vi "配置变量_temp_赋值.vi"(8 "error in (no error)":errorcluster caption="错误输入（无错误）") -> (0 "error out":errorcluster caption="错误输出")   [LabVIEW 2014]
doc: "该模板用于创建子VI。"
uses:
  glb/glb_data.vi
  R/manifest.vi
  glb/glb_static.vi
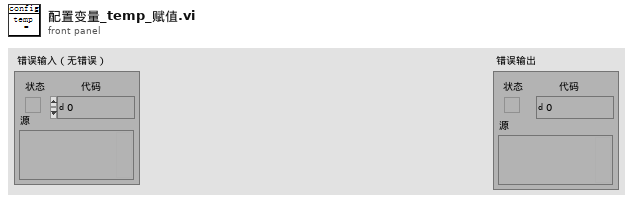
[diagram p1: front panel]
types:
  T1 = cluster{"控制型号":string, "插槽数目":u32, "板卡信息":cluster{"板卡类型":string, "信号类型":string, "上限":string, "下限":string, "单位":string, "通道数":u32, "最大采样率":u32, "设置采样率":u32, "附加条件":string[], "板卡型号":string}[]}
  T2 = cluster{"侧边栏数据":cluster{"来源":string, "名称":string}[], "界面刷间隔率":dbl}
  T3 = cluster{"名称":string, "简称":string, "单位":string, "附加":string[], "类型":enum16{"测试模块", "FPGA", "cRIO", "其他设备", "总体展示"}}[]
  T4 = cluster{"应用状态":bool, "vi名称":string, "刷新间隔":u32, "显示数据精度":u32, "储存数据精度":u32}[]
  T5 = cluster{"应用1":string[], "应用2":string[], "应用3":string[], "应用4":string[], "应用5":string[], "应用6":string[], "应用7":string[], "应用8":string[], "分母":cluster{"来源":string, "名称":string}, "加":cluster{"来源":string, "名称":string}[], "减":cluster{"来源":string, "名称":string}[]}
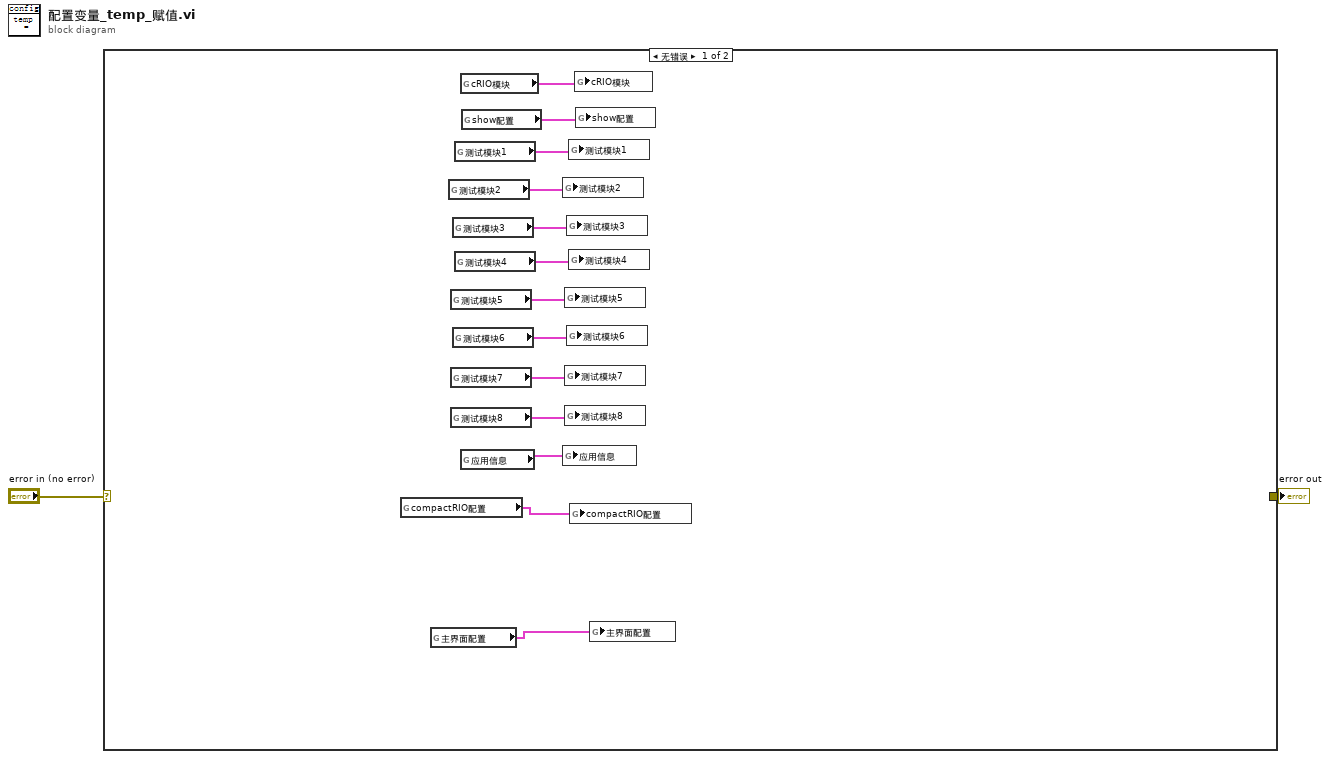
[diagram p0: block diagram]
diagram:
  n1 = case shown="无错误" "error in (no error)" {
    selector: "error in (no error)" -> [_ w16]
    tunnel: [_ w16] -> w1
    frame No Error {
      n2 = global read "glb_static.vi" "compactRIO配置"() -> (w4:T1)
      n3 = global read "glb_static.vi" "主界面配置"() -> (w3:T2)
      n4 = global read "glb_data.vi" "测试模块2"() -> (w8:T3)
      n5 = global read "glb_data.vi" "测试模块5"() -> (w11:T3)
      n6 = global read "glb_data.vi" "测试模块7"() -> (w13:T3)
      n7 = global read "glb_data.vi" "测试模块8"() -> (w14:T3)
      n8 = global read "glb_data.vi" "测试模块3"() -> (w9:T3)
      n9 = global read "glb_data.vi" "测试模块6"() -> (w12:T3)
      n10 = global read "glb_data.vi" "测试模块1"() -> (w7:T3)
      n11 = global read "glb_data.vi" "测试模块4"() -> (w10:T3)
      n12 = global read "glb_data.vi" "cRIO模块"() -> (w5:T3)
      n13 = global read "manifest.vi" "应用信息"() -> (w15:T4)
      n14 = global read "glb_data.vi" "show配置"() -> (w6:T5)
      n15 = global write "配置变量_temp.vi" "测试模块2"(w8) -> ()
      n16 = global write "配置变量_temp.vi" "应用信息"(w15) -> ()
      n17 = global write "配置变量_temp.vi" "测试模块5"(w11) -> ()
      n18 = global write "配置变量_temp.vi" "测试模块7"(w13) -> ()
      n19 = global write "配置变量_temp.vi" "测试模块8"(w14) -> ()
      n20 = global write "配置变量_temp.vi" "测试模块3"(w9) -> ()
      n21 = global write "配置变量_temp.vi" "测试模块6"(w12) -> ()
      n22 = global write "配置变量_temp.vi" "测试模块1"(w7) -> ()
      n23 = global write "配置变量_temp.vi" "测试模块4"(w10) -> ()
      n24 = global write "配置变量_temp.vi" "compactRIO配置"(w4) -> ()
      n25 = global write "配置变量_temp.vi" "cRIO模块"(w5) -> ()
      n26 = global write "配置变量_temp.vi" "show配置"(w6) -> ()
      n27 = global write "配置变量_temp.vi" "主界面配置"(w3) -> ()
    }
    frame Error {
    }
  }
  "error out" <- w1
